vi "Simulator2.vi"() -> ()   [LabVIEW 2014]
panel:
  out "Output":dbl format="%#_13g"
  out "path":path
  in  "Input":dbl format="%#_13g"
  in  "Action":string
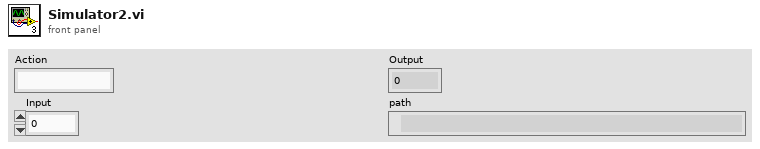
[diagram p1: front panel]
types:
  T1 = enum16{"open", "replace", "create", "open or create", "replace or create", "replace or create with confirmation"}
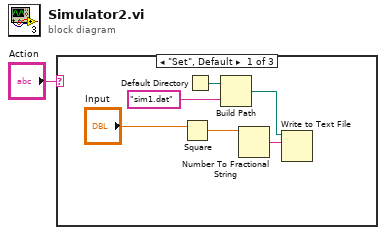
[diagram p0: block diagram]
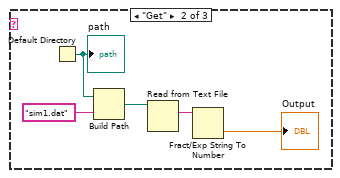
[diagram p2: hidden frame]
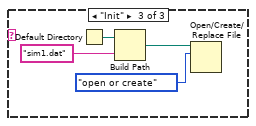
[diagram p3: hidden frame]
diagram:
  n1 = case shown="\"Set\", Default" "Action" {
    frame "Set", Default {
      n2 = Square(x="Input") -> (x^2=w3:dbl)
      n3 = Default Directory() -> (w4:path)
      n4 = Build Path(base path=w4, name or relative path="sim1.dat") -> (appended path=w6:path)
      n5 = Number To Fractional String(number=w3) -> (F-format string=w5:string)  [unwired: 3 in]
      n6 = Write to Text File(file (use dialog)=w6, text=w5) -> ()  [unwired: 2 in, 3 out]
    }
    frame "Get" {
      n7 = Default Directory() -> (w9:path)
      "path" <- w9
      n8 = Build Path(base path=w9, name or relative path="sim1.dat") -> (appended path=w11:path)
      n9 = Read from Text File(file (use dialog)=w11) -> (text=w10:string)  [unwired: 3 in, 3 out]
      n10 = Fract/Exp String To Number(string=w10) -> (number=→"Output":dbl)  [unwired: 3 in, 1 out]
    }
    frame "Init" {
      n11 = Default Directory() -> (w13:path)
      n12 = Build Path(base path=w13, name or relative path="sim1.dat") -> (appended path=w15:path)
      n13 = Open/Create/Replace File(file path (use dialog)=w15, operation (0:open)=T1."open or create") -> ()  [unwired: 4 in, 3 out]
    }
  }
